vi "http connection handler.vi"(9 "remote address":string, 10 "server properties":T1={"max url size"=8000, "max header"=8000, "timeout ms"=5000, "max data size"=104857600}, 11 "connection":refnum<k5>) -> ()   [LabVIEW 2013]
uses:
  http server properties.ctl
  http parse state.ctl
  http request.ctl
  http method.ctl
  http response.ctl
  http response packet type.ctl
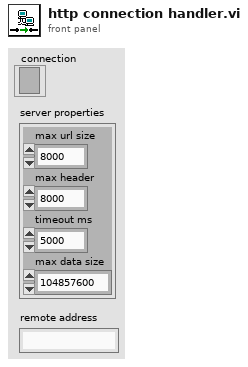
[diagram p1: front panel]
types:
  T1 = typedef "http server properties.ctl" = cluster{"max url size":i32, "max header":i32, "timeout ms":i32, "max data size":i32}
  T2 = typedef "http response.ctl" = cluster{"packet type":T3, "version":string, "reason code":u16, "status string":string, "header dictionary":variant, "cookies":string[], "data":string}
  T3 = typedef "http response packet type.ctl" = enum16{"full response", "header only", "data only", "last data"}
  T4 = typedef "http request.ctl" = cluster{"remote address":string, "method":T5, "target":string, "version":string, "header dictionary":variant, "data":string, "has data?":bool}
  T5 = typedef "http method.ctl" = enum16{"GET", "POST", "PUT", "DELETE", "HEAD", "OPTIONS"}
  T6 = typedef "http parse state.ctl" = enum16{"function", "headers", "data"}
  T7 = enum16{"Standard", "Buffered", "CRLF", "Immediate"}
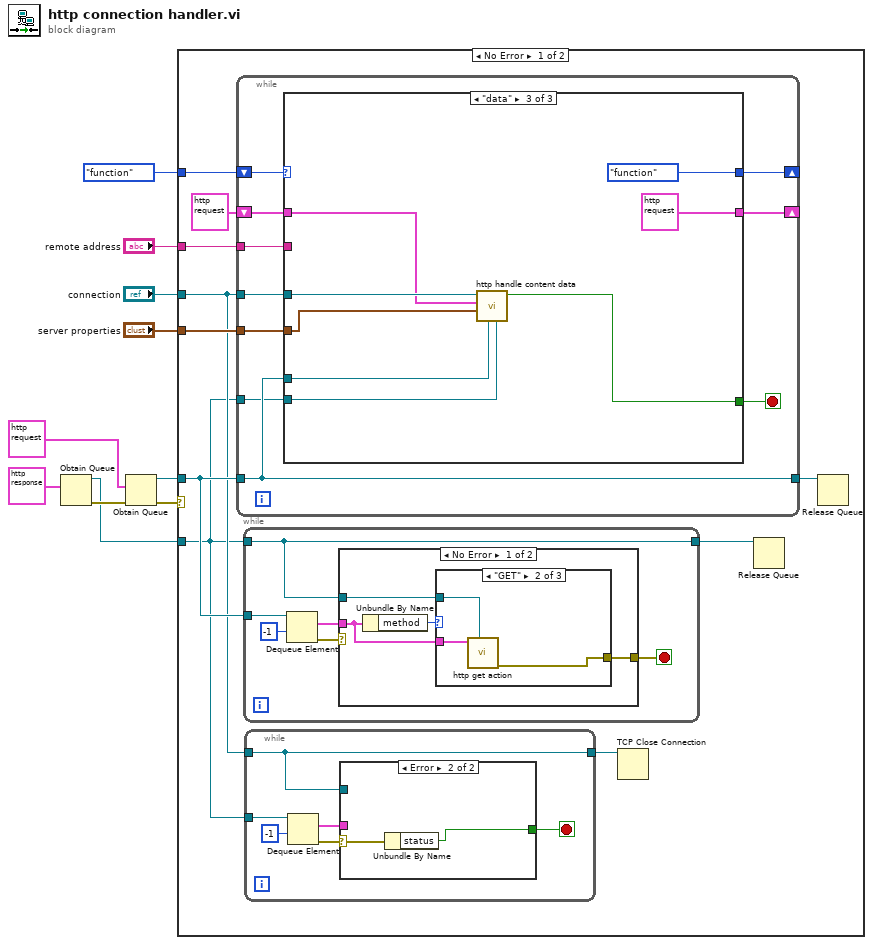
[diagram p0: block diagram]
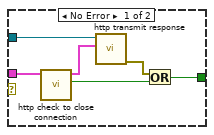
[diagram p2: hidden frame]
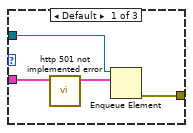
[diagram p3: hidden frame]
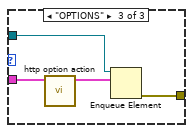
[diagram p4: hidden frame]
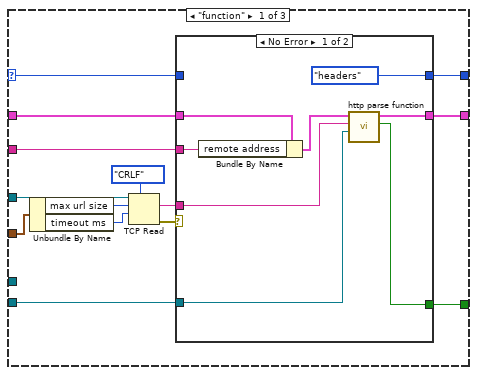
[diagram p6: hidden frame]
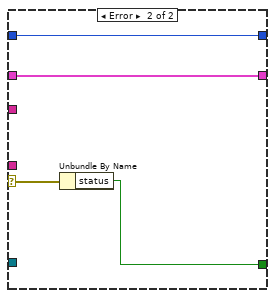
[diagram p7: hidden frame]
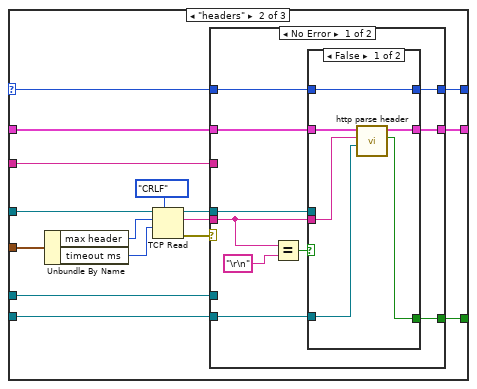
[diagram p8: hidden frame]
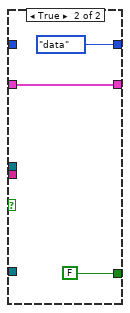
[diagram p9: hidden frame]
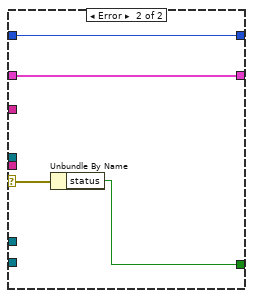
[diagram p10: hidden frame]
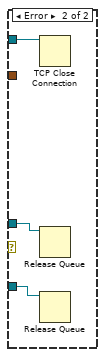
[diagram p11: hidden frame]
diagram:
  n1 = Obtain Queue(element data type=T2 {"packet type"=enum."full response", "version"="", "reason code"=0, "status string"="", "header dictionary"=variant, "cookies"=[], "data"=""} ("application request")) -> (queue out=w2:refnum<queue>, error out=w4:errorcluster)  [unwired: 4 in, 1 out]
  n2 = Obtain Queue(element data type=T4 {"remote address"="", "method"=enum."GET", "target"="", "version"="", "header dictionary"=variant, "data"="", "has data?"=FALSE} ("application request"), error in (no error)=w4) -> (queue out=w6:refnum<queue>, error out=w7:errorcluster)  [unwired: 3 in, 1 out]
  n3 = case shown="No Error" w7 {
    tunnel: http_parse_state."function" -> [w20 _]
    tunnel: "connection" -> [w12 w142]
    tunnel: "remote address" -> [w19 _]
    tunnel: w6 -> [w16 w141]
    tunnel: "server properties" -> [w15 _]
    tunnel: w2 -> [w11 w140]
    frame No Error {
      n4 = while {
        tunnel: w12 -> [w64]
        shift-right: [w65] -> _
        shift-left: T4 {"remote address"="", "method"=enum."GET", "target"="", "version"="", "header dictionary"=variant(cluster{"key":string, "value":string}[] []), "data"="", "has data?"=FALSE} ("application request") -> [w66]
        tunnel: w16 -> [w60]
        shift-right: [w63] -> _
        shift-left: w20 -> [w57]
        tunnel: w19 -> [w61]
        tunnel: [w60] -> w17
        tunnel: w15 -> [w59]
        tunnel: w11 -> [w58]
        stop <- w62 stop-if-true
        n5 = case shown="\"data\"" w57 {
          selector: w57 -> [w70 w96 _]
          tunnel: w66 -> [w80 w108 w135]
          tunnel: [w79 w107 T4 {"remote address"="", "method"=enum."GET", "target"="", "version"="", "header dictionary"=variant(cluster{"key":string, "value":string}[] []), "data"="", "has data?"=FALSE} ("application request")] -> w65
          tunnel: w64 -> [w76 w104 w136]
          tunnel: [w74 w102 http_parse_state."function"] -> w63
          tunnel: [w73 w101 w137] -> w62
          tunnel: w61 -> [w72 w99 _]
          tunnel: w60 -> [_ w98 w133]
          tunnel: w59 -> [w69 w95 w134]
          tunnel: w58 -> [w71 w97 w132]
          frame "function" {
            n6 = Unbundle By Name(w69) -> ("max url size"=w68:i32, "timeout ms"=w67:i32)
            n7 = TCP Read(connection ID=w76, bytes to read=w68, 7:T7."CRLF" ("mode (standard)"), 9:w67) -> (data out=w75:string, error out=w77:errorcluster)  [unwired: 1 in, 1 out]
            n8 = case shown="No Error" w77 {
              selector: w77 -> [_ w91]
              tunnel: w80 -> [w85 w92]
              tunnel: [w86 w92] -> w79
              tunnel: [w84 w89] -> w73
              tunnel: w75 -> [w88 _]
              tunnel: w70 -> [_ w90]
              tunnel: [http_parse_state."headers" w90] -> w74
              tunnel: w72 -> [w83 _]
              tunnel: w71 -> [w82 _]
              frame No Error {
                n9 = Bundle By Name(cluster=w85, "remote address"=w83) -> (w81:T4)
                n10 = call "http parse function.vi"("transmit queue"=w82, "data in"=w88, "application request in"=w81) -> ("abort"=w84:bool, "application request out"=w86:T4)  [unwired: 7 in]
              }
              frame Error {
                n11 = Unbundle By Name(w91) -> ("status"=w89:bool)
              }
            }
          }
          frame "headers" {
            n12 = Unbundle By Name(w95) -> ("max header"=w94:i32, "timeout ms"=w93:i32)
            n13 = TCP Read(connection ID=w104, bytes to read=w94, 7:T7."CRLF" ("mode (standard)"), 9:w93) -> (connection ID out=w100:refnum<k5>, data out=w103:string, error out=w105:errorcluster)  [unwired: 1 in]
            n14 = case shown="No Error" w105 {
              selector: w105 -> [_ w130]
              tunnel: w108 -> [w114 w131]
              tunnel: [w115 w131] -> w107
              tunnel: [w113 w128] -> w101
              tunnel: w98 -> [_ _]
              tunnel: w103 -> [w117 _]
              tunnel: w96 -> [w118 w129]
              tunnel: [w116 w129] -> w102
              tunnel: w100 -> [w112 _]
              tunnel: w99 -> [_ _]
              tunnel: w97 -> [w111 _]
              frame No Error {
                n15 = Equal?(x=w117, y="\r\n" ("x")) -> (x = y?=w109:bool)
                n16 = case shown="False" w109 {
                  tunnel: w117 -> [w123 _]
                  tunnel: w114 -> [w122 w126]
                  tunnel: [w121 w126] -> w115
                  tunnel: w118 -> [w124 _]
                  tunnel: [w124 http_parse_state."data"] -> w116
                  tunnel: [w120 FALSE ("abort")] -> w113
                  tunnel: w112 -> [_ _]
                  tunnel: w111 -> [w119 _]
                  frame False {
                    n17 = call "http parse header.vi"("transmit queue"=w119, "data in"=w123, "application request"=w122) -> ("abort"=w120:bool, "application request out"=w121:T4)  [unwired: 7 in]
                  }
                  frame True {
                  }
                }
              }
              frame Error {
                n18 = Unbundle By Name(w130) -> ("status"=w128:bool)
              }
            }
          }
          frame "data" {
            n19 = call "http handle content data.vi"("transmit queue"=w132, "exec queue"=w133, "server properties"=w134, "application request"=w135, "TCP Network Connection in"=w136) -> ("abort"=w137:bool)  [unwired: 6 in]
          }
        }
      }
      n20 = while {
        tunnel: w11 -> [w35]
        tunnel: [w35] -> w14
        tunnel: w16 -> [w40]
        stop <- w37 stop-if-true
        n21 = Dequeue Element(queue=w40, timeout in ms (-1)=-1) -> (element=w36:T4, error out=w38:errorcluster)  [unwired: 1 in, 2 out]
        n22 = case shown="No Error" w38 {
          selector: w38 -> [_ w56]
          tunnel: [w42 w56] -> w37
          tunnel: w36 -> [w43 _]
          tunnel: w35 -> [w41 _]
          frame No Error {
            n23 = Unbundle By Name(w43) -> ("method"=w44:T5)
            n24 = case shown="\"GET\"" w44 {
              tunnel: w43 -> [w48 w51 w55]
              tunnel: [w47 w50 w53] -> w42
              tunnel: w41 -> [w46 w49 w52]
              frame Default {
                n25 = call "http 501 not implemented error.vi"("application request in"=w48) -> ("application request out"=w45:T2)  [unwired: 10 in]
                n26 = Enqueue Element(queue=w46, element=w45) -> (error out=w47:errorcluster)  [unwired: 2 in, 2 out]
              }
              frame "GET" {
                n27 = call "http get action.vi"("transmit queue"=w49, "application request in"=w51) -> ("connection error"=w50:errorcluster)  [unwired: 9 in]
              }
              frame "OPTIONS" {
                n28 = call "http option action.vi"("application request in"=w55) -> ("application request out"=w54:T2)  [unwired: 10 in]
                n29 = Enqueue Element(queue=w52, element=w54) -> (error out=w53:errorcluster)  [unwired: 2 in, 2 out]
              }
            }
          }
          frame Error {
          }
        }
      }
      n30 = while {
        tunnel: w12 -> [w21]
        tunnel: [w21] -> w13
        tunnel: w11 -> [w26]
        stop <- w23 stop-if-true
        n31 = Dequeue Element(queue=w26, timeout in ms (-1)=-1) -> (element=w22:T2, error out=w24:errorcluster)  [unwired: 1 in, 2 out]
        n32 = case shown="Error" w24 {
          selector: w24 -> [_ w34]
          tunnel: [w31 w33] -> w23
          tunnel: w22 -> [w29 _]
          tunnel: w21 -> [w32 _]
          frame No Error {
            n33 = call "http check to close connection.vi"("application request"=w29) -> ("close connection?"=w27:bool, "application request out"=w28:T2)  [unwired: 9 in]
            n34 = call "http transmit response.vi"("application request"=w28, "tcp connection"=w32) -> ("error out"=w30:errorcluster)  [unwired: 9 in]
            n35 = Or(x=w30, y=w27) -> (x .or. y?=w31:bool)
          }
          frame Error {
            n36 = Unbundle By Name(w34) -> ("status"=w33:bool)
          }
        }
      }
      n37 = TCP Close Connection(connection ID=w13) -> ()  [unwired: 2 in, 2 out]
      n38 = Release Queue(queue=w14) -> ()  [unwired: 2 in, 3 out]
      n39 = Release Queue(queue=w17) -> ()  [unwired: 2 in, 3 out]
    }
    frame Error {
      n40 = TCP Close Connection(connection ID=w142) -> ()  [unwired: 2 in, 2 out]
      n41 = Release Queue(queue=w141) -> ()  [unwired: 2 in, 3 out]
      n42 = Release Queue(queue=w140) -> ()  [unwired: 2 in, 3 out]
    }
  }
